vi "Simulated Error.vi"(8 "error in (no error)":errorcluster, 11 "Controls in":refnum<class "Controls.lvclass">) -> (0 "error out":errorcluster, 3 "Controls out":refnum<class "Controls.lvclass">)   [LabVIEW 2020, in "Controls.lvlib" / "Controls.lvclass"]
uses:
  Controls.lvclass
  Controls.lvclass/Controls.ctl
  <vilib>/ErrorRing/Error Ring.xnode
  <vilib>/Utility/error.llb/Error Cluster From Error Code.vi
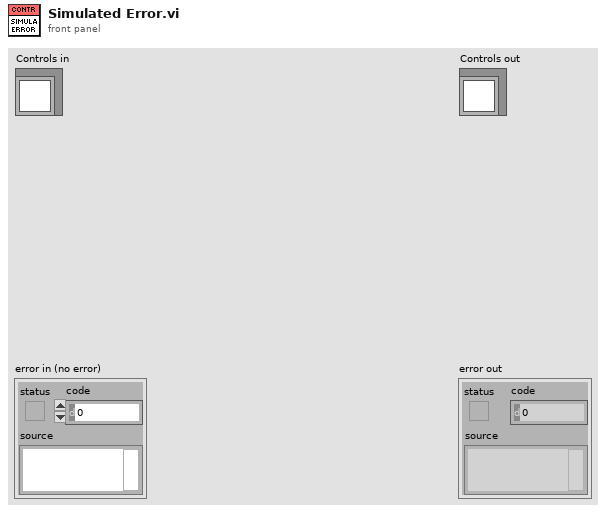
[diagram p1: front panel]
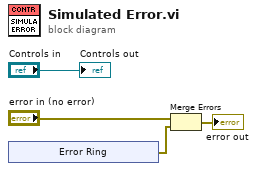
[diagram p0: block diagram]
diagram:
  n1 = xnode "Error Ring"() -> ("error out"=w1:errorcluster)
  n2 = Merge Errors("error in (no error)", w1) -> (→"error out":errorcluster)
  "Controls out" <- "Controls in"
